vi "Get factors-test harness.vi"() -> ()   [LabVIEW 2021, in "Numeric Utilities.lvlib"]
uses:
  Numeric Utilities.lvlib
  Named Timers/Named Timers.lvlib
panel:
  out "Loop iteration":i32
  out "Elapsed time (ms)":u32
  # "Test vector 1\nLabVIEW: 6 ms\nPython: between 0.5 and 1 ms \n\nTest  vector 2\nLabVIEW: 64 ms\nPython: 11 ms"
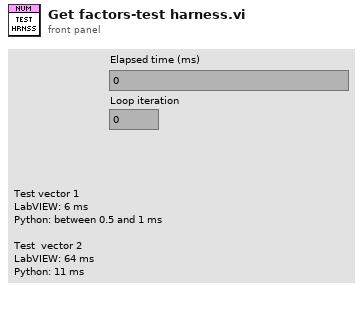
[diagram p1: front panel]
types:
  T1 = typedef "Numeric Utilities.lvlib/Factors cluster.ctl" = cluster{"Factor":i32, "Power":i32}
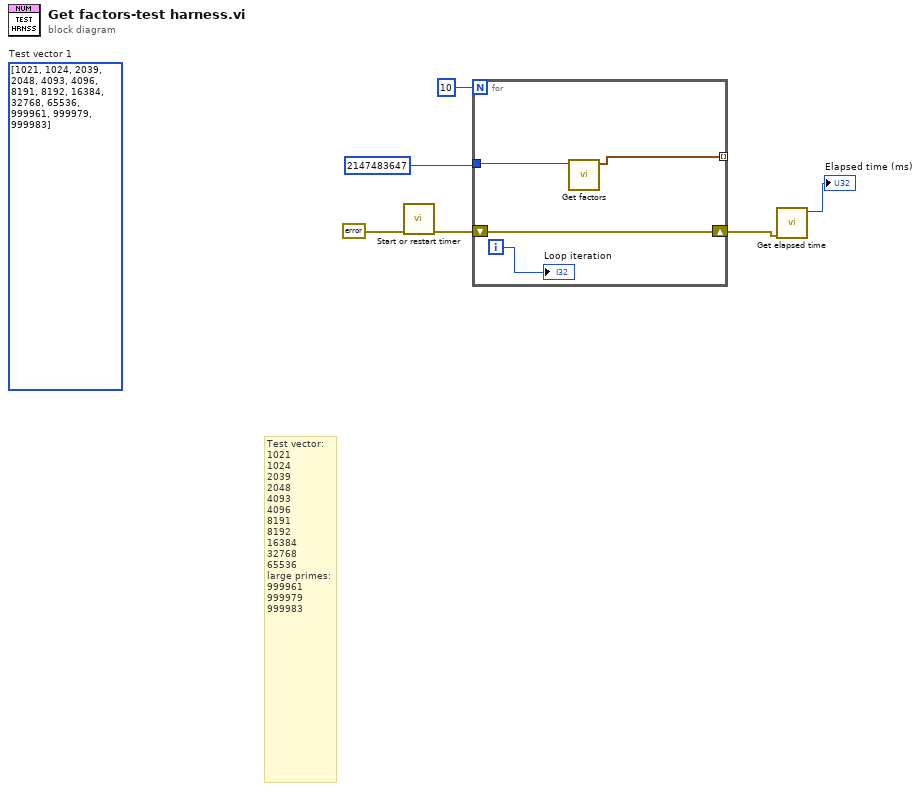
[diagram p0: block diagram]
diagram:
  (unwired) i32[] [1021, 1024, 2039, 2048, 4093, 4096, 8191, 8192, 16384, 32768, 65536, 999961, 999979, 999983]  # Test vector 1
  # "Test vector:\n1021\n1024\n2039\n2048\n4093\n4096\n8191\n8192\n16384\n32768\n65536\nlarge primes:\n999961\n999979\n999983"
  n1 = call "Start or restart timer.vi"("error in (no error)"=errorcluster {"status"=FALSE, "code"=0, "source"=""} ("error constant")) -> ("error out"=w5:errorcluster)  [unwired: 10 in]
  n2 = for {
    N: 10 -> [_]
    tunnel: [w10] -> _ mode=indexing
    shift-right: [w9] -> w4
    shift-left: w5 -> [w9]
    tunnel: 2147483647 -> [w8]
    i -> [w7]
    n3 = call "Get factors.vi"("x"=w8) -> ("Factors out"=w10:T1[])  [unwired: 5 in, 5 out]
    "Loop iteration" <- w7
  }
  n4 = call "Get elapsed time.vi"("error in (no error)"=w4) -> ("Elapsed time (ms)"=→"Elapsed time (ms)":u32)  [unwired: 7 in, 3 out]
